vi "Pockels Cal-Objective setup handler.vi"   [LabVIEW 2013]
uses:
  Globals/gl_Calibration globals.vi
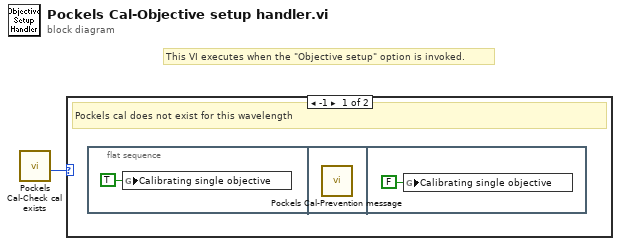
[diagram p0: block diagram]
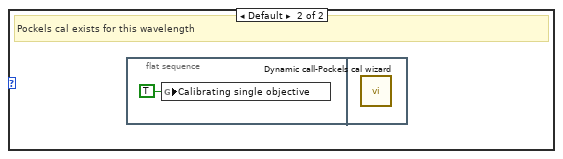
[diagram p2: hidden frame]
diagram:
  # "This VI executes when the \"Objective setup\" option is invoked."
  n1 = call "Pockels Cal-Check cal exists.vi"() -> ("-1 if Pockels cal does not exist"=w1:i32)  [unwired: 11 in]
  n2 = case shown="-1" w1 {
    frame -1 {
      # "Pockels cal does not exist for this wavelength"
      n3 = flat-sequence {
        frame #0 {
          n4 = global write "gl_Calibration globals.vi" "Calibrating single objective"(TRUE ("Calibrating single objective")) -> ()
        }
        frame #1 {
          n5 = call "Pockels Cal-Prevention message.vi"() -> ()  [unwired: 11 in, 1 out]
        }
        frame #2 {
          n6 = global write "gl_Calibration globals.vi" "Calibrating single objective"(FALSE ("Calibrating single objective")) -> ()
        }
      }
    }
    frame Default {
      # "Pockels cal exists for this wavelength"
      n7 = flat-sequence {
        frame #0 {
          n8 = global write "gl_Calibration globals.vi" "Calibrating single objective"(TRUE ("Calibrating single objective")) -> ()
        }
        frame #1 {
          n9 = call "Dynamic call-Pockels cal wizard.vi"() -> ()  [unwired: 11 in, 1 out]
        }
      }
    }
  }
